vi "Motion Profile Drive.vi"(8 "error in (no error)":errorcluster, 9 "Right Buffer name":string="Auto", 10 "Left Buffer name":string="Auto", 11 "CTRE Drive in":refnum<class "CTRE Drive.lvclass">) -> (0 "error out":errorcluster, 3 "CTRE Drive out":refnum<class "CTRE Drive.lvclass">)   [LabVIEW 2019, in "Drive.lvlib" / "CTRE Drive.lvclass"]
doc: "switches into motion profiling"
uses:
  CTRE Drive.lvclass
  Tank Drive.lvclass
  <vilib>/Rock Robotics/WPI/ThirdParty/Phoenix-LabVIEW/Motor Controller/Controls/CTRE_Phoenix_MotorControl_MotionProfileControlMode.ctl
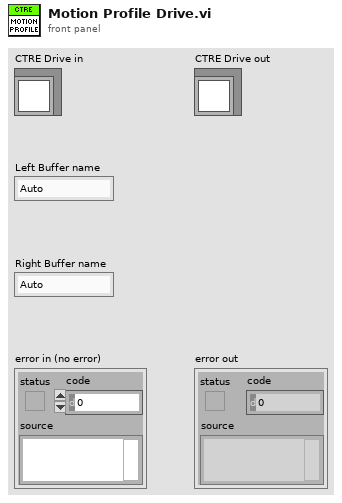
[diagram p1: front panel]
types:
  T1 = typedef "CTRE_Phoenix_MotorControl_MotionProfileControlMode.ctl" = u16
  T2 = typedef "Drive.lvlib/Tank Drive.lvclass/Motor Controller Names.ctl" = cluster{"Left Lead":string, "Right Lead":string, "Left Followers":string[], "Right Followers":string[]}
  T3 = typedef "CTRE_Phoenix_MotorControl_BufferedTrajectoryPointStream_DeviceRef.ctl" = cluster{"Handle":u64, "Library Path":path}
  T4 = typedef "WPI_MotorControlDeviceRef.ctl" = cluster{"DeviceStatus":errorcluster, "Type":T5, "PWM":cluster{"PWM Channel":T6, "DeadBand":T7}, "CAN":cluster{"Device Number":u8, "SetOutput VI Ref":variant, "GetOutput VI Ref":variant, "Enable VI Ref":variant, "Disable VI Ref":variant, "Data":variant}, "Invert":bool, "DIO PWM":cluster{"PWM \"Enable\" Channel":T6, "DIOChannel":T8, "PWM Rate":dbl}}
  T5 = typedef "WPI_MotorControlType.ctl" = enum16{"PWM", "CAN", "DIO PWM"}
  T6 = typedef "FPGA_DIOPWMChannel.ctl" = enum8{"PWM 0", "PWM 1", "PWM 2", "PWM 3", "PWM 4", "PWM 5", "PWM 6", "PWM 7", "PWM 8", "PWM 9", "PWM MXP 0", "PWM MXP 1", "PWM MXP 2", "PWM MXP 3", "PWM MXP 4", "PWM MXP 5", "PWM MXP 6", "PWM MXP 7", "PWM MXP 8", "PWM MXP 9", "Invalid"}
  T7 = typedef "WPI_PWMDeadband.ctl" = cluster{"Name":string, "maxPositivePwm":i32, "minPositivePwm":i32, "centerPwm":i32, "maxNegativePwm":i32, "minNegativePwm":i32, "angularRange":u16}
  T8 = typedef "FPGA_DIOChannel.ctl" = enum8{"DIO 0", "DIO 1", "DIO 2", "DIO 3", "DIO 4", "DIO 5", "DIO 6", "DIO 7", "DIO 8", "DIO 9", "DIO MXP 0", "DIO MXP 1", "DIO MXP 2", "DIO MXP 3", "DIO MXP 4", "DIO MXP 5", "DIO MXP 6", "DIO MXP 7", "DIO MXP 8", "DIO MXP 9", "DIO MXP 10", "DIO MXP 11", "DIO MXP 12", "DIO MXP 13", "DIO MXP 14", "DIO MXP 15", "SPI Port CS1", "SPI Port CS2", "SPI Port CS3", "SPI Port MISO", "SPI Port MOSI", "Invalid"}
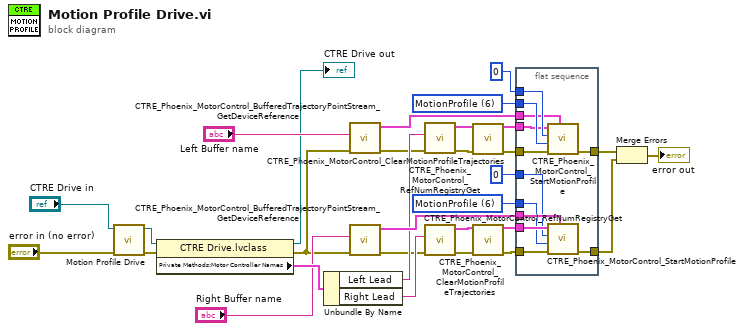
[diagram p0: block diagram]
diagram:
  w14 = T1 6 items=["MotionProfile"=6, "MotionProfileArc"=10] ("Control Mode")
  w29 = T1 6 items=["MotionProfile"=6, "MotionProfileArc"=10] ("Control Mode")
  n1 = call-parent "Motion Profile Drive.vi"("error in (no error)"="error in (no error)", "Tank Drive in"="CTRE Drive in") -> ("error out"=w5:errorcluster, "Tank Drive out"=w7:refnum<class "CTRE Drive.lvclass">)  [unwired: 8 in]
  n2 = property class="CTRE Drive.lvclass"(reference=w7, error in=w5) -> (reference out=→"CTRE Drive out":refnum<class "CTRE Drive.lvclass">, error out=w3:errorcluster, "Private Methods:Motor Controller Names"=w30:T2)
  n3 = Unbundle By Name(w30) -> ("Left Lead"=w12:string, "Right Lead"=w13:string)
  n4 = call <vilib>:"CTRE_Phoenix_MotorControl_BufferedTrajectoryPointStream_GetDeviceReference.vi"("error in (no error)"=w3, "refnum name"="Left Buffer name") -> ("error out"=w2:errorcluster, "BufferedTrajectoryPointStream_DevRef"=w26:T3)  [unwired: 8 in]
  n5 = call <vilib>:"CTRE_Phoenix_MotorControl_BufferedTrajectoryPointStream_GetDeviceReference.vi"("error in (no error)"=w3, "refnum name"="Right Buffer name") -> ("error out"=w1:errorcluster, "BufferedTrajectoryPointStream_DevRef"=w17:T3)  [unwired: 8 in]
  n6 = call <vilib>:"CTRE_Phoenix_MotorControl_RefNumRegistryGet.vi"("error in (no error)"=w2, "refnum name"=w12) -> ("error out"=w23:errorcluster, "PhoenixMotorControlDevRef"=w27:T4)  [unwired: 8 in]
  n7 = call <vilib>:"CTRE_Phoenix_MotorControl_RefNumRegistryGet.vi"("error in (no error)"=w1, "refnum name"=w13) -> ("error out"=w20:errorcluster, "PhoenixMotorControlDevRef"=w16:T4)  [unwired: 8 in]
  n8 = call <vilib>:"CTRE_Phoenix_MotorControl_ClearMotionProfileTrajectories.vi"("PhoenixMotorControlDevRef"=w27, "error in"=w23) -> ("PhoenixMotorControlDevRef"=w24:T4, "error out"=w22:errorcluster)  [unwired: 12 in]
  n9 = call <vilib>:"CTRE_Phoenix_MotorControl_ClearMotionProfileTrajectories.vi"("PhoenixMotorControlDevRef"=w16, "error in"=w20) -> ("PhoenixMotorControlDevRef"=w19:T4, "error out"=w21:errorcluster)  [unwired: 12 in]
  n10 = flat-sequence {
    tunnel: w29 -> [w42]
    tunnel: u32 0 ("minBufferedPts") -> [w41]
    tunnel: w26 -> [w40]
    tunnel: w24 -> [w39]
    tunnel: w22 -> [w38]
    tunnel: w21 -> [w37]
    tunnel: w19 -> [w36]
    tunnel: w17 -> [w35]
    tunnel: u32 0 ("minBufferedPts") -> [w34]
    tunnel: w14 -> [w33]
    tunnel: [w32] -> w11
    tunnel: [w31] -> w10
    frame #0 {
      n11 = call <vilib>:"CTRE_Phoenix_MotorControl_StartMotionProfile.vi"("BufferedTrajectoryPointStream_DevRef"=w40, "error in"=w38, "Control Mode"=w42, "minBufferedPts"=w41, "PhoenixMotorControlDevRef"=w39) -> ("error out"=w32:errorcluster)  [unwired: 5 in, 1 out]
      n12 = call <vilib>:"CTRE_Phoenix_MotorControl_StartMotionProfile.vi"("BufferedTrajectoryPointStream_DevRef"=w35, "error in"=w37, "Control Mode"=w33, "minBufferedPts"=w34, "PhoenixMotorControlDevRef"=w36) -> ("error out"=w31:errorcluster)  [unwired: 5 in, 1 out]
    }
  }
  n13 = Merge Errors(w11, w10) -> (→"error out":errorcluster)
